vi "Enable Lockstep.vi"(7 "Lockstep Group (1)":u8=1, 8 "error in (no error)":errorcluster, 9 "Device Number":string, 10 "Axis Numbers (1,2)":i32[](array[numeric])=[1, 2], 11 "VISA resource name":refnum<visa-resource-name>) -> (0 "error out":errorcluster, 3 "VISA resource name out":refnum<visa-resource-name>)   [LabVIEW 2015, in "Zaber A Series.lvlib"]
doc: "Enables lockstep mode on a device that supports it. Lockstep mode groups two or more axes and moves them in unison, preserving the relative offset that was between them when lockstep mode was enabled. \n\nTo configure a lockstep group you must specify a number for the group, between 1 and the value of the \"lockstep.numgroups\" device setting. The group number must not be already in use. You must also specify at least two axis numbers to be members of the group, and none of the axes may already be members of a group.\n\nNormal move commands do not work on axes that are part of a lockstep group; once you have enabled lockstep you must use lockstep-specific VIs until after disabling lockstep. Lockstep mode persists across device resets and power cycles.\n\nThis VI does not check in advance for error conditions such as lockstep not being supported on the device or no group numbers being available.\n\nThis VI requires that the Initialize VI has been called with the same serial port."
uses:
  Zaber A Series.lvlib
  Private/All Commands.ctl
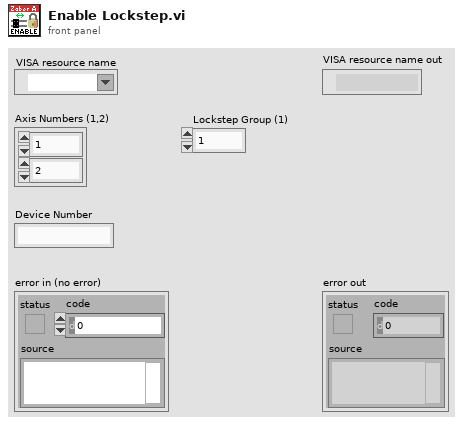
[diagram p1: front panel]
types:
  T1 = typedef "Zaber A Series.lvlib/All Commands.ctl" = string
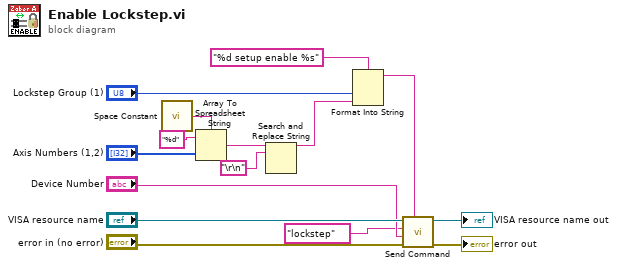
[diagram p0: block diagram]
diagram:
  n1 = call <vilib>:"Space Constant.vi"() -> ("String"=w13:string)
  n2 = Array To Spreadsheet String(delimiter (Tab)=w13, array="Axis Numbers (1,2)", 3:"%d" ("format string")) -> (spreadsheet string=w11:string)
  n3 = Search and Replace String(input string=w11, search string="\r\n") -> (result string=w3:string)  [unwired: 6 in, 3 out]
  n4 = Format Into String(format string="%d setup enable %s", "Lockstep Group (1)", w3) -> (resulting string=w5:string)  [unwired: 2 in, 1 out]
  n5 = call "Send Command.vi"("Data"=w5, "error in (no error)"="error in (no error)", "Device and Axis"="Device Number", "Command"=T1 "lockstep" ("Complete Command List"), "VISA resource name"="VISA resource name") -> ("error out"=→"error out":errorcluster, "VISA resource name out"=→"VISA resource name out":refnum<visa-resource-name>)  [unwired: 1 in, 4 out]
